vi "Show FrontPanel.vi"(7 "Front Panel Title":string, 8 "error in (no error)":errorcluster, 10 "SubPanel ref":refnum<vi>, 11 "Parallel Process in":refnum<class "Parallel Process.lvclass">) -> (0 "error out":errorcluster, 3 "Parallel Process out":refnum<class "Parallel Process.lvclass">)   [LabVIEW 2011, in "Messenging.lvlib" / "Parallel Process.lvclass"]
uses:
  Parallel Process.lvclass
  Parallel Process.lvclass/Parallel Process.ctl
panel:
  # "Opens Front Panel (optionally opens it in a subPanel)"
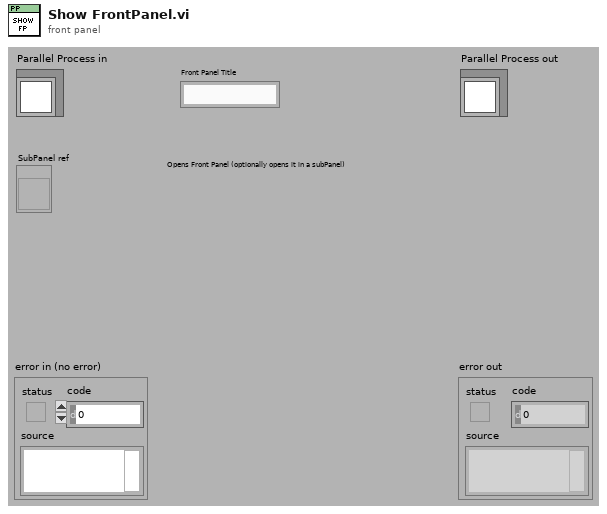
[diagram p1: front panel]
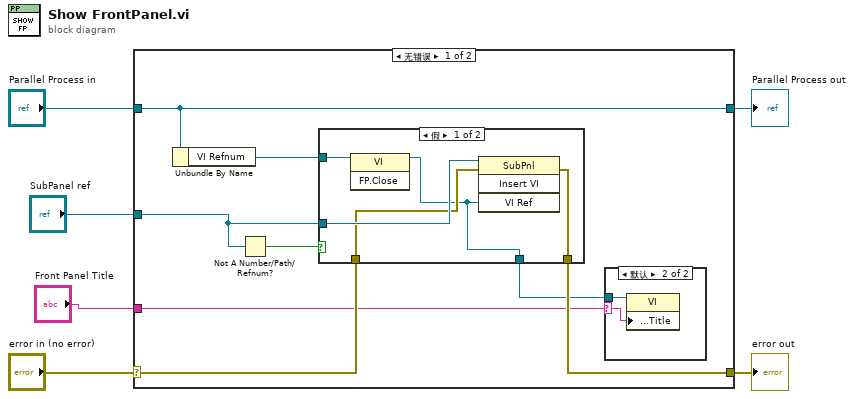
[diagram p0: block diagram]
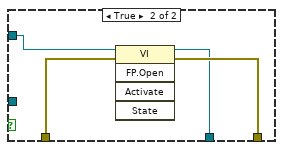
[diagram p3: hidden frame]
diagram:
  n1 = case shown="无错误" "error in (no error)" {
    selector: "error in (no error)" -> [w13 w27]
    tunnel: [w12 w27] -> w5
    tunnel: [w14 w26] -> w3
    tunnel: "Parallel Process in" -> [w14 w26]
    tunnel: "SubPanel ref" -> [w9 _]
    tunnel: "Front Panel Title" -> [w8 _]
    frame No Error {
      n2 = Unbundle By Name(w14) -> ("VI Refnum"=w11:refnum<vi>)
      n3 = Not A Number/Path/Refnum?(number/path/refnum=w9) -> (NaN/Path/Refnum?=w10:bool)
      n4 = case shown="假" w10 {
        tunnel: w13 -> [w18 w24]
        tunnel: [w21 w23] -> w12
        tunnel: w11 -> [w20 w25]
        tunnel: w9 -> [w19 _]
        tunnel: [w17 w22] -> w7
        frame False {
          n5 = invoke class="VI" method="FP.Close"(reference=w20) -> (reference out=w17:refnum<vi>)  [unwired: 2 in, 2 out]
          n6 = invoke class="SubPnl" method="Insert VI"(reference=w19, error in=w18, "VI Ref"=w17) -> (error out=w21:errorcluster)  [unwired: 1 in, 3 out]
        }
        frame True {
          n7 = invoke class="VI" method="FP.Open"(reference=w25, error in=w24) -> (reference out=w22:refnum<vi>, error out=w23:errorcluster)  [unwired: 3 in, 3 out]
        }
      }
      n8 = case shown="默认" w8 {
        selector: w8 -> [_ w15]
        tunnel: w7 -> [_ w16]
        frame "" {
        }
        frame Default {
          n9 = property class="VI"(reference=w16, "Front Panel.Title"=w15) -> ()  [unwired: 1 in, 2 out]
        }
      }
    }
    frame Error {
    }
  }
  "error out" <- w5
  "Parallel Process out" <- w3
